vi "2DVectorNormalizer.vi"() -> ()   [LabVIEW 2016]
panel:
  out "2D vector 2":dbl[](array[numeric])
  in  "2D vector":dbl[](array[numeric])
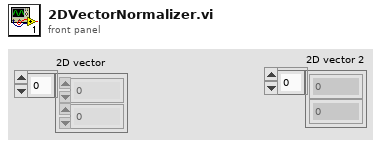
[diagram p1: front panel]
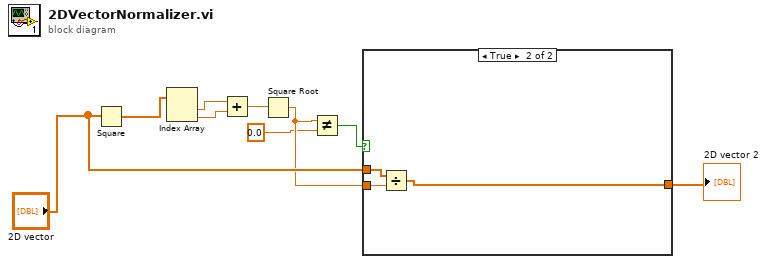
[diagram p0: block diagram]
diagram:
  n1 = Square(x="2D vector") -> (x^2=w9:dbl[])
  n2 = Index Array(array=w9) -> (element #1=w8:dbl, element #2=w7:dbl)  [unwired: 2 in]
  n3 = Add(x=w8, y=w7) -> (x+y=w6:dbl)
  n4 = Square Root(x=w6) -> (sqrt(x)=w4:dbl)
  n5 = Not Equal?(x=w4, y=0.0) -> (x != y?=w2:bool)
  n6 = case shown="True" w2 {
    tunnel: "2D vector" -> [w10 w13]
    tunnel: w4 -> [_ w12]
    tunnel: [w10 w11] -> w1
    frame False {
    }
    frame True {
      n7 = Divide(x=w13, y=w12) -> (x/y=w11:dbl[])
    }
  }
  "2D vector 2" <- w1
